vi "WS1050_NI6501_Relay_Control_manual.vi"(4 "Ring":u16(ring) items=["All Off", "Bank 1", "Bank 2", "Bank 3"], 11 "error in (no error)":errorcluster, 14 "Relay_ 10":bool) -> (0 "RF_SWitch_Ctrl1":bool, 1 "RF_SWitch_Ctrl3":bool, 2 "RL_3_SW_PIC":bool, 3 "RF_SWitch_Ctrl6":bool, 5 "RF_SWitch_Ctrl2":bool, 7 "RL_1_SW_PIC":bool, 9 "RL_2_SW_PIC":bool, 12 "RF_SWitch_Ctrl4":bool, 13 "RF_SWitch_Ctrl5":bool, 15 "error out":errorcluster)   [LabVIEW 2009]
doc: "I. Description:\nThis example demonstrates how to write values to a digital output channel.\n\nII. Instructions for Running:\n1. Select the digital lines on the DAQ device to be written.\n2. Select a value to write.\nNote: The array control is sized for 8 lines, if using a different amount of lines, change the number of elements in the array to equal the number of lines chosen.\n\nIII. Block Diagram Steps:\n1. Create a Digital Output channel. Use one channel for all lines. You can alternatively use one channel for each line, but then use a different polymorphic version of the DAQmx Write VI.\n2. Call the Start VI to start the task.\n3. Write the digital Boolean array data in a loop until the user hits the stop button or an error occurs. This write VI writes a single sample of digital data on demand, so no timeout is necessary.\n4. Call the Clear Task VI to clear the Task.\n5. Use the popup dialog box to display an error or warning if any.\n\nIV. I/O Connections Overview:\nMake sure your signal output terminals match the Lines I/O Control. In this case wire the item to receive the signal to the first eight digital lines on your DAQ Device."
uses:
  <vilib>/DAQmx/write.llb/DAQmx Write (Digital Bool 1Line 1Point).vi
  <vilib>/DAQmx/create/channels.llb/DAQmx Create Channel (DO-Digital Output).vi
panel:
  in  "Lines 10":tag="Dev2/port1/line2" caption="Lines"
  in  "Lines 9":tag="Dev2/port1/line4" caption="Lines"
  in  "Lines 8":tag="Dev2/port2/line7" caption="Lines"
  in  "Lines 7":tag="Dev2/port2/line6" caption="Lines"
  in  "Lines 6":tag="Dev2/port2/line5" caption="Lines"
  in  "Lines 5":tag="Dev2/port2/line4" caption="Lines"
  in  "Lines 4":tag="Dev2/port2/line3" caption="Lines"
  in  "Lines 3":tag="Dev2/port2/line2" caption="Lines"
  in  "Lines 2":tag="Dev2/port2/line1" caption="Lines"
  in  "Lines":tag="Dev2/port2/line0"
  # "For instructions, select Help>>Show Context Help"
  # "Channel Parameters"
  # "Pin 11"
  # "Pin 14"
  # "Pin16"
  # "Line 5"
  # "Line 2"
  # "Line 0"
  # "Pin 09"
  # "Pin 13"
  # "Pin 15"
  # "Line 7"
  # "Line 3"
  # "Line 1"
  # "Pin 6"
  # "Pin 10"
  # "Pin 12"
  # "Line 4 Port1"
  # "Line 6"
  # "Line 4"
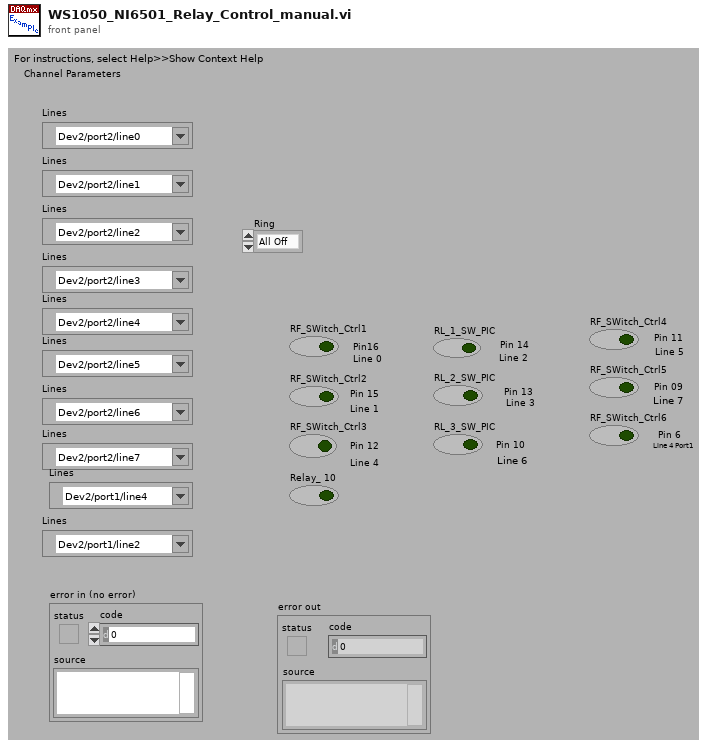
[diagram p1: front panel]
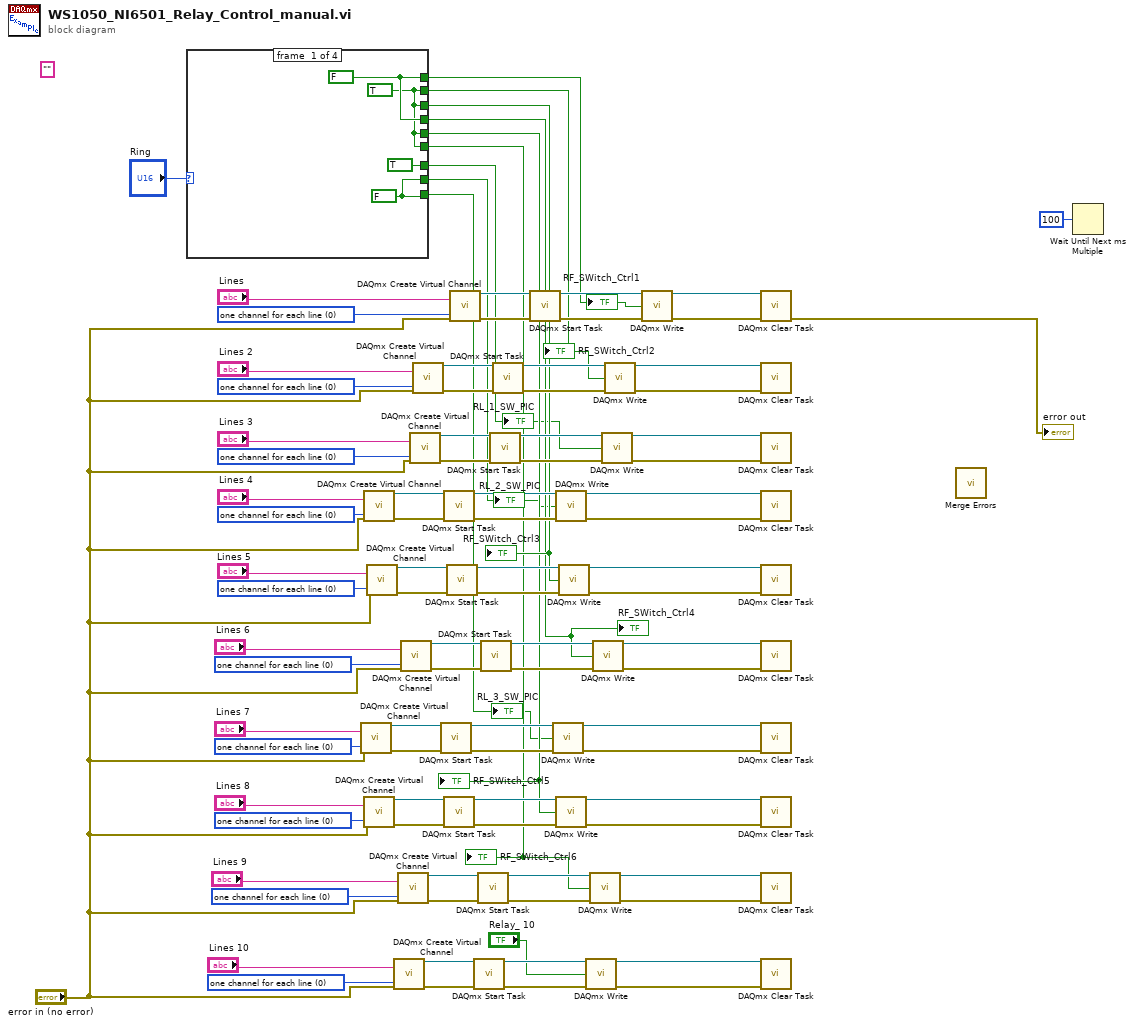
[diagram p0: block diagram]
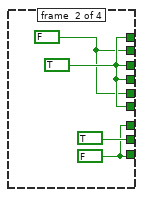
[diagram p2: hidden frame]
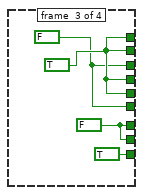
[diagram p3: hidden frame]
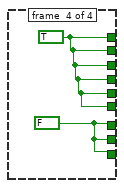
[diagram p4: hidden frame]
diagram:
  (unwired) ""
  w21 = 0 items=["one channel for each line", "one channel for all lines"] ("line grouping")
  w22 = 0 items=["one channel for each line", "one channel for all lines"] ("line grouping")
  w37 = 0 items=["one channel for each line", "one channel for all lines"] ("line grouping")
  w38 = 0 items=["one channel for each line", "one channel for all lines"] ("line grouping")
  w69 = 0 items=["one channel for each line", "one channel for all lines"] ("line grouping")
  w54 = 0 items=["one channel for each line", "one channel for all lines"] ("line grouping")
  w53 = 0 items=["one channel for each line", "one channel for all lines"] ("line grouping")
  w70 = 0 items=["one channel for each line", "one channel for all lines"] ("line grouping")
  w85 = 0 items=["one channel for each line", "one channel for all lines"] ("line grouping")
  w87 = 0 items=["one channel for each line", "one channel for all lines"] ("line grouping")
  n1 = case shown="3" "Ring" {
    tunnel: [w98 w102 w104 w108] -> w11
    tunnel: [w97 w101 w104 w108] -> w10
    tunnel: [w97 w102 w103 w108] -> w9
    tunnel: [w98 w102 w104 w108] -> w8
    tunnel: [w97 w101 w104 w108] -> w7
    tunnel: [w97 w102 w103 w108] -> w6
    tunnel: [TRUE ("RF_SWitch_Ctrl1") w99 w106 w107] -> w5
    tunnel: [w95 TRUE ("RF_SWitch_Ctrl1") w106 w107] -> w4
    tunnel: [w95 w99 TRUE ("RF_SWitch_Ctrl1") w107] -> w3
    frame #0 {
      w95 = FALSE ("RF_SWitch_Ctrl1")
      w97 = TRUE ("RF_SWitch_Ctrl1")
      w98 = FALSE ("RF_SWitch_Ctrl1")
    }
    frame #1 {
      w99 = FALSE ("RF_SWitch_Ctrl1")
      w102 = TRUE ("RF_SWitch_Ctrl1")
      w101 = FALSE ("RF_SWitch_Ctrl1")
    }
    frame #2 {
      w106 = FALSE ("RF_SWitch_Ctrl1")
      w104 = TRUE ("RF_SWitch_Ctrl1")
      w103 = FALSE ("RF_SWitch_Ctrl1")
    }
    frame #3 {
      w108 = TRUE ("RF_SWitch_Ctrl1")
      w107 = FALSE ("RF_SWitch_Ctrl1")
    }
  }
  "RF_SWitch_Ctrl1" <- w11
  "RF_SWitch_Ctrl2" <- w10
  "RL_1_SW_PIC" <- w5
  "RF_SWitch_Ctrl3" <- w9
  "RL_2_SW_PIC" <- w4
  "RF_SWitch_Ctrl4" <- w8
  "RF_SWitch_Ctrl5" <- w7
  "RL_3_SW_PIC" <- w3
  "RF_SWitch_Ctrl6" <- w6
  n2 = call-poly <vilib>:"DAQmx Create Virtual Channel.vi"("lines"="Lines 7", "line grouping"=w22, "error in"="error in (no error)") -> ("task out"=w25:refnum<k21>, "error out"=w24:errorcluster)  [unwired: 11 in]
  n3 = call-poly <vilib>:"DAQmx Create Virtual Channel.vi"("lines"="Lines 4", "line grouping"=w69, "error in"="error in (no error)") -> ("task out"=w66:refnum<k21>, "error out"=w67:errorcluster)  [unwired: 11 in]
  n4 = call-poly <vilib>:"DAQmx Create Virtual Channel.vi"("lines"="Lines 8", "line grouping"=w37, "error in"="error in (no error)") -> ("task out"=w34:refnum<k21>, "error out"=w35:errorcluster)  [unwired: 11 in]
  n5 = call-poly <vilib>:"DAQmx Create Virtual Channel.vi"("lines"="Lines 5", "line grouping"=w54, "error in"="error in (no error)") -> ("task out"=w57:refnum<k21>, "error out"=w56:errorcluster)  [unwired: 11 in]
  n6 = call-poly <vilib>:"DAQmx Create Virtual Channel.vi"("lines"="Lines 10", "line grouping"=w21, "error in"="error in (no error)") -> ("task out"=w18:refnum<k21>, "error out"=w19:errorcluster)  [unwired: 11 in]
  n7 = call-poly <vilib>:"DAQmx Create Virtual Channel.vi"("lines"="Lines 9", "line grouping"=w38, "error in"="error in (no error)") -> ("task out"=w41:refnum<k21>, "error out"=w40:errorcluster)  [unwired: 11 in]
  n8 = call-poly <vilib>:"DAQmx Create Virtual Channel.vi"("lines"="Lines 6", "line grouping"=w53, "error in"="error in (no error)") -> ("task out"=w50:refnum<k21>, "error out"=w51:errorcluster)  [unwired: 11 in]
  n9 = call-poly <vilib>:"DAQmx Create Virtual Channel.vi"("lines"="Lines 3", "line grouping"=w70, "error in"="error in (no error)") -> ("task out"=w73:refnum<k21>, "error out"=w72:errorcluster)  [unwired: 11 in]
  n10 = call-poly <vilib>:"DAQmx Create Virtual Channel.vi"("lines"="Lines 2", "line grouping"=w85, "error in"="error in (no error)") -> ("task out"=w82:refnum<k21>, "error out"=w83:errorcluster)  [unwired: 11 in]
  n11 = call <vilib>:"DAQmx Start Task.vi"("task/channels in"=w25, "error in"=w24) -> ("task out"=w27:refnum<k21>, "error out"=w29:errorcluster)  [unwired: 12 in]
  n12 = call <vilib>:"DAQmx Start Task.vi"("task/channels in"=w66, "error in"=w67) -> ("task out"=w64:refnum<k21>, "error out"=w62:errorcluster)  [unwired: 12 in]
  n13 = call <vilib>:"DAQmx Start Task.vi"("task/channels in"=w34, "error in"=w35) -> ("task out"=w32:refnum<k21>, "error out"=w30:errorcluster)  [unwired: 12 in]
  n14 = call <vilib>:"DAQmx Start Task.vi"("task/channels in"=w57, "error in"=w56) -> ("task out"=w59:refnum<k21>, "error out"=w61:errorcluster)  [unwired: 12 in]
  n15 = call-poly <vilib>:"DAQmx Create Virtual Channel.vi"("lines"="Lines", "line grouping"=w87, "error in"="error in (no error)") -> ("task out"=w90:refnum<k21>, "error out"=w89:errorcluster)  [unwired: 11 in]
  n16 = call <vilib>:"DAQmx Start Task.vi"("task/channels in"=w18, "error in"=w19) -> ("task out"=w16:refnum<k21>, "error out"=w14:errorcluster)  [unwired: 12 in]
  n17 = call <vilib>:"DAQmx Start Task.vi"("task/channels in"=w41, "error in"=w40) -> ("task out"=w43:refnum<k21>, "error out"=w45:errorcluster)  [unwired: 12 in]
  n18 = call <vilib>:"DAQmx Start Task.vi"("task/channels in"=w50, "error in"=w51) -> ("task out"=w48:refnum<k21>, "error out"=w46:errorcluster)  [unwired: 12 in]
  n19 = call <vilib>:"DAQmx Start Task.vi"("task/channels in"=w73, "error in"=w72) -> ("task out"=w75:refnum<k21>, "error out"=w77:errorcluster)  [unwired: 12 in]
  n20 = call <vilib>:"DAQmx Start Task.vi"("task/channels in"=w82, "error in"=w83) -> ("task out"=w80:refnum<k21>, "error out"=w78:errorcluster)  [unwired: 12 in]
  n21 = call <vilib>:"DAQmx Start Task.vi"("task/channels in"=w90, "error in"=w89) -> ("task out"=w92:refnum<k21>, "error out"=w94:errorcluster)  [unwired: 12 in]
  n22 = call-poly <vilib>:"DAQmx Write.vi"("task/channels in"=w27, "data"=w3, "error in"=w29) -> ("task out"=w26:refnum<k21>, "error out"=w28:errorcluster)  [unwired: 10 in, 1 out]
  n23 = call-poly <vilib>:"DAQmx Write.vi"("task/channels in"=w64, "data"=w4, "error in"=w62) -> ("task out"=w65:refnum<k21>, "error out"=w63:errorcluster)  [unwired: 10 in, 1 out]
  n24 = call-poly <vilib>:"DAQmx Write.vi"("task/channels in"=w32, "data"=w7, "error in"=w30) -> ("task out"=w33:refnum<k21>, "error out"=w31:errorcluster)  [unwired: 10 in, 1 out]
  n25 = call-poly <vilib>:"DAQmx Write.vi"("task/channels in"=w59, "data"=w9, "error in"=w61) -> ("task out"=w58:refnum<k21>, "error out"=w60:errorcluster)  [unwired: 10 in, 1 out]
  n26 = call-poly <vilib>:"DAQmx Write.vi"("task/channels in"=w16, "data"="Relay_ 10", "error in"=w14) -> ("task out"=w17:refnum<k21>, "error out"=w15:errorcluster)  [unwired: 10 in, 1 out]
  n27 = call-poly <vilib>:"DAQmx Write.vi"("task/channels in"=w43, "data"=w6, "error in"=w45) -> ("task out"=w42:refnum<k21>, "error out"=w44:errorcluster)  [unwired: 10 in, 1 out]
  n28 = call-poly <vilib>:"DAQmx Write.vi"("task/channels in"=w48, "data"=w8, "error in"=w46) -> ("task out"=w49:refnum<k21>, "error out"=w47:errorcluster)  [unwired: 10 in, 1 out]
  n29 = call-poly <vilib>:"DAQmx Write.vi"("task/channels in"=w75, "data"=w5, "error in"=w77) -> ("task out"=w74:refnum<k21>, "error out"=w76:errorcluster)  [unwired: 10 in, 1 out]
  n30 = call-poly <vilib>:"DAQmx Write.vi"("task/channels in"=w80, "data"=w10, "error in"=w78) -> ("task out"=w81:refnum<k21>, "error out"=w79:errorcluster)  [unwired: 10 in, 1 out]
  n31 = call-poly <vilib>:"DAQmx Write.vi"("task/channels in"=w92, "data"=w11, "error in"=w94) -> ("task out"=w91:refnum<k21>, "error out"=w93:errorcluster)  [unwired: 10 in, 1 out]
  n32 = call <vilib>:"DAQmx Clear Task.vi"("task in"=w91, "error in"=w93) -> ("error out"=→"error out":errorcluster)  [unwired: 13 in]
  n33 = call <vilib>:"DAQmx Clear Task.vi"("task in"=w81, "error in"=w79) -> ()  [unwired: 13 in, 1 out]
  n34 = call <vilib>:"DAQmx Clear Task.vi"("task in"=w74, "error in"=w76) -> ()  [unwired: 13 in, 1 out]
  n35 = call <vilib>:"DAQmx Clear Task.vi"("task in"=w65, "error in"=w63) -> ()  [unwired: 13 in, 1 out]
  n36 = call <vilib>:"DAQmx Clear Task.vi"("task in"=w58, "error in"=w60) -> ()  [unwired: 13 in, 1 out]
  n37 = call <vilib>:"DAQmx Clear Task.vi"("task in"=w49, "error in"=w47) -> ()  [unwired: 13 in, 1 out]
  n38 = call <vilib>:"DAQmx Clear Task.vi"("task in"=w26, "error in"=w28) -> ()  [unwired: 13 in, 1 out]
  n39 = call <vilib>:"DAQmx Clear Task.vi"("task in"=w33, "error in"=w31) -> ()  [unwired: 13 in, 1 out]
  n40 = call <vilib>:"DAQmx Clear Task.vi"("task in"=w42, "error in"=w44) -> ()  [unwired: 13 in, 1 out]
  n41 = call <vilib>:"DAQmx Clear Task.vi"("task in"=w17, "error in"=w15) -> ()  [unwired: 13 in, 1 out]
  n42 = call <vilib>:"Merge Errors.vi"() -> ()  [unwired: 7 in, 1 out]
  n43 = Wait Until Next ms Multiple(millisecond multiple=u32 100 ("milliseconds to wait")) -> ()  [unwired: 1 out]
